vi "Update_data.vi"(8 "input data":variant, 9 "condition":string, 10 "table":string, 11 "columns":string[](array[string])) -> (0 "connection reference out":T1, 1 "Application Directory":path, 2 "connection information":path, 3 "error out":errorcluster)   [LabVIEW 2014]
doc: "Update data where condition applies"
uses:
  <vilib>/addons/database/Connection.llb/Conn ObjectReference.ctl
  <vilib>/addons/database/Connection.llb/DB Tools Open Connec (Path).vi
  <vilib>/addons/database/NI_Database_API.lvlib
panel:
  # "Update Database Data"
  # "Outputs"
  # "Inputs"
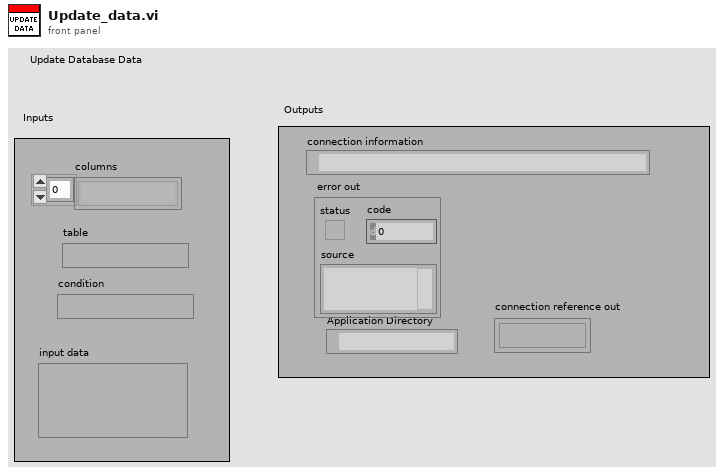
[diagram p1: front panel]
types:
  T1 = typedef "NI_Database_API.lvlib/Conn ObjectReference.ctl" = refnum<k1>
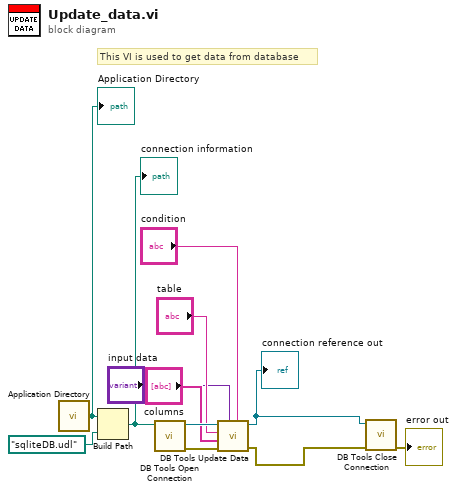
[diagram p0: block diagram]
diagram:
  # "This VI is used to get data from database"
  n1 = call <vilib>:"Application Directory.vi"() -> ("Application Directory"=w10:path)
  "Application Directory" <- w10
  n2 = Build Path(base path=w10, name or relative path=path "sqliteDB.udl" ("connection information")) -> (appended path=w9:path)
  "connection information" <- w9
  n3 = call-poly <vilib>:"DB Tools Open Connection.vi"("connection information"=w9) -> ("error out"=w11:errorcluster, "connection reference"=w12:T1)  [unwired: 7 in]
  n4 = call <vilib>:"DB Tools Update Data.vi"("condition"="condition", "data"="input data", "error in (no error)"=w11, "columns"="columns", "table"="table", "connection reference"=w12) -> ("error out"=w3:errorcluster, "connection reference out"=w4:T1)  [unwired: 4 in]
  "connection reference out" <- w4
  n5 = call <vilib>:"DB Tools Close Connection.vi"("error in (no error)"=w3, "connection reference"=w4) -> ("error out"=→"error out":errorcluster)  [unwired: 5 in]
